vi "adjust.vi"(8 "error in (no error)":errorcluster, 11 "YK090623DAQmxAnalogDetector in":refnum<class "DetectorYK090623DAQmxAnalog.lvclass">) -> (0 "error out":errorcluster, 3 "YK090623DAQmxAnalogDetector out":refnum<class "DetectorYK090623DAQmxAnalog.lvclass">)   [LabVIEW 2011, in "DetectorYK090623DAQmxAnalog.lvclass"]
uses:
  DetectorYK090623DAQmxAnalog.lvclass
  DetectorYK090623DAQmxAnalog.lvclass/DetectorYK090623DAQmxAnalog.ctl
  AnalogOut/AnalogOutDL101207DAQmx/AnalogOutDL101207DAQmx/AnalogOutDL101207DAQmx.lvclass
  common/classes/ErrorController/ErrorController/class_data.vi
  common/classes/ErrorController/ErrorController/ErrorController.lvclass
panel:
  in  "done button":bool
  in  "output voltage":dbl[unit](slide) scale=0.0..2.0
  # "Adjust detector gain"
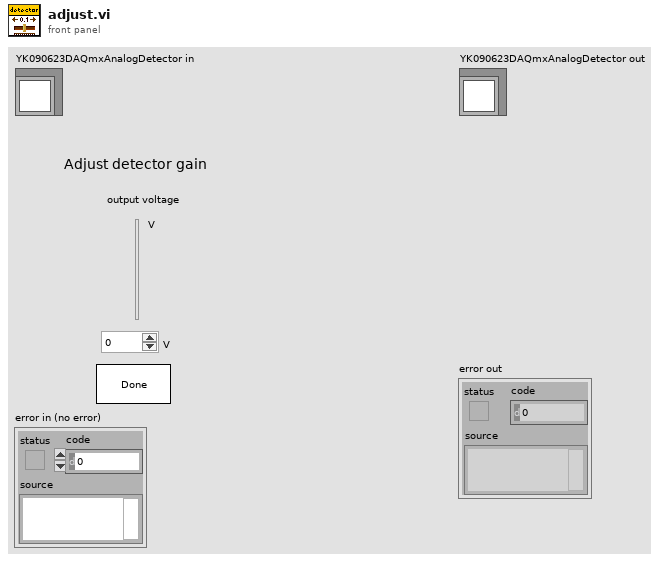
[diagram p1: front panel]
types:
  T1 = typedef "GenericDetector.lvclass/status_enum.ctl" = enum16{"disabled", "enabled"}
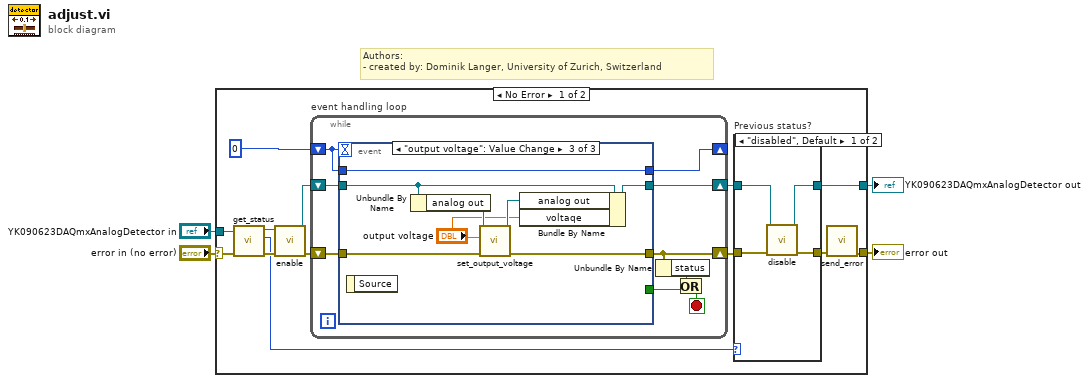
[diagram p0: block diagram]
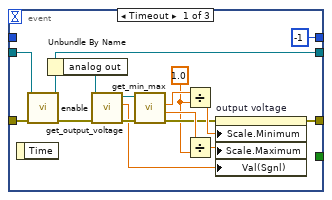
[diagram p3: hidden frame]
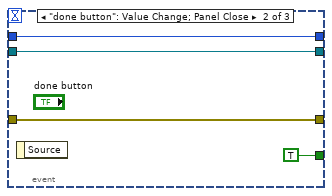
[diagram p4: hidden frame]
diagram:
  # "Authors: \n- created by: Dominik Langer, University of Zurich, Switzerland"
  n1 = case shown="No Error" "error in (no error)" {
    selector: "error in (no error)" -> [w16 w62]
    tunnel: [w6 w62] -> w3
    tunnel: [w7 w61] -> w1
    tunnel: "YK090623DAQmxAnalogDetector in" -> [w15 w61]
    frame No Error {
      n2 = call-dynamic "get_status.vi"("error in (no error)"=w16, "GenericEmissionSensor.lvclass in"=w15) -> ("error out"=w14:errorcluster, "status"=w10:T1, "GenericEmissionSensor.lvclass out"=w12:refnum<class "DetectorYK090623DAQmxAnalog.lvclass">)  [unwired: 7 out]
      n3 = call-dynamic "enable.vi"("error in (no error)"=w14, "GenericEmissionSensor in"=w12) -> ("error out"=w13:errorcluster, "GenericEmissionSensor out"=w11:refnum<class "DetectorYK090623DAQmxAnalog.lvclass">)  [unwired: 8 out]
      n4 = while "event handling loop" {
        shift-right: [w28] -> w8
        shift-left: w11 -> [w32]
        shift-right: [w29] -> _
        shift-left: 0 -> [w30]
        shift-right: [w27] -> w9
        shift-left: w13 -> [w31]
        stop <- w24 stop-if-true
        n5 = event shown="[2] \"output voltage\": Value Change" {
          selector: _ -> [_ _ _]
          dyn-events: _ -> [_ _ _]
          timeout: w30 -> [_ _ _]
          tunnel: w32 -> [w34 w52 w55]
          tunnel: [w33 w52 w54] -> w28
          tunnel: w31 -> [w36 w50 w60]
          tunnel: [_ TRUE _] -> w26
          tunnel: [w47 w50 w59] -> w27
          tunnel: w30 -> [_ w49 w53]
          tunnel: [-1 w49 w53] -> w29
          event Timeout {
            w38 = dbl[unit] 1.0 ("y")
            n6 = event-data() -> ()  [unwired: 2 out]
            n7 = call-dynamic "enable.vi"("error in (no error)"=w36, "GenericEmissionSensor in"=w34) -> ("error out"=w35:errorcluster, "GenericEmissionSensor out"=w33:refnum<class "DetectorYK090623DAQmxAnalog.lvclass">)  [unwired: 8 out]
            n8 = Unbundle By Name(w33) -> ("analog out"=w39:refnum<class "AnalogOutDL101207DAQmx.lvclass">)
            n9 = call-dynamic "get_output_voltage.vi"("error in (no error)"=w35, "DAQmxAnalogOut.lvclass in"=w39) -> ("error out"=w41:errorcluster, "current voltage"=w37:dbl[unit], "DAQmxAnalogOut.lvclass out"=w40:refnum<class "AnalogOutDL101207DAQmx.lvclass">)  [unwired: 7 in]
            n10 = call-dynamic "get_min_max.vi"("error in (no error)"=w41, "DAQmxAnalogOut.lvclass in"=w40) -> ("error out"=w42:errorcluster, "maximum"=w44:dbl[unit], "minimum"=w46:dbl[unit])  [unwired: 6 in, 1 out]
            n11 = Divide(x=w46, y=w38) -> (x/y=w45:dbl)
            n12 = Divide(x=w44, y=w38) -> (x/y=w43:dbl)
            n13 = property on="output voltage" class="Slide (strict)"(error in=w42, "Scale.Minimum"=w45, "Scale.Maximum"=w43, "Val(Sgnl)"=w37) -> (error out=w47:errorcluster)  [unwired: 1 in, 1 out]
          }
          event "done button": Value Change; Panel Close {
            n14 = event-data() -> ()  [unwired: 2 out]
          }
          event "output voltage": Value Change {
            n15 = event-data() -> ()  [unwired: 2 out]
            n16 = Unbundle By Name(w55) -> ("analog out"=w58:refnum<class "AnalogOutDL101207DAQmx.lvclass">)
            n17 = call-dynamic "set_output_voltage.vi"("error in (no error)"=w60, "output value"="output voltage", "DAQmxAnalogOut in"=w58) -> ("error out"=w59:errorcluster, "DAQmxAnalogOut out"=w57:refnum<class "AnalogOutDL101207DAQmx.lvclass">)  [unwired: 7 in]
            n18 = Bundle By Name(cluster=w55, "analog out"=w57, "voltaqe"="output voltage") -> (w54:refnum<class "DetectorYK090623DAQmxAnalog.lvclass">)
          }
        }
        n19 = Unbundle By Name(w27) -> ("status"=w25:bool)
        n20 = Or(x=w25, y=w26) -> (x .or. y?=w24:bool)
      }
      n21 = case "Previous status?" shown="\"disabled\", Default" w10 {
        tunnel: w9 -> [w21 w22]
        tunnel: w8 -> [w19 w23]
        tunnel: [w20 w22] -> w5
        tunnel: [w18 w23] -> w7
        frame "disabled", Default {
          n22 = call-dynamic "disable.vi"("error in (no error)"=w21, "GenericEmissionSensor in"=w19) -> ("error out"=w20:errorcluster, "GenericEmissionSensor out"=w18:refnum<class "DetectorYK090623DAQmxAnalog.lvclass">)  [unwired: 8 out]
        }
        frame "enabled" {
        }
      }
      n23 = call "send_error.vi"("error in (no error)"=w5) -> ("error out"=w6:errorcluster)  [unwired: 10 in]
    }
    frame Error {
    }
  }
  "error out" <- w3
  "YK090623DAQmxAnalogDetector out" <- w1
